vi "Lockin.DAQ.Create Sample Clock.vi"(8 "error in (no error)":errorcluster, 11 "Lockin.DAQ":refnum<class "Instrument.DAQ.lvclass">) -> (0 "error out":errorcluster, 3 "Lockin.DAQ":refnum<class "Instrument.DAQ.lvclass">)   [LabVIEW 2019, in "Instrument.DAQ.lvclass"]
uses:
  Instrument.DAQ.lvclass
  Instrument.DAQ.lvclass/Instrument.DAQ.ctl
  <vilib>/DAQmx/configure/timing.llb/DAQmx Timing (Sample Clock).vi
  <resource>/objmgr/daqmx.rc
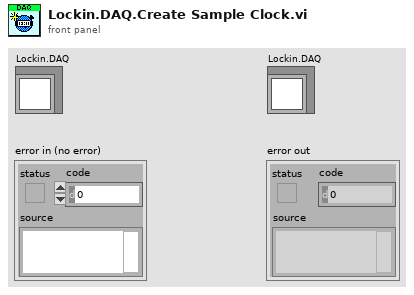
[diagram p1: front panel]
types:
  T1 = typedef "Instrument.DAQ.lvclass/DAQType-enum.ctl" = enum16{"None", "USB 4431", "PXI 446x"}
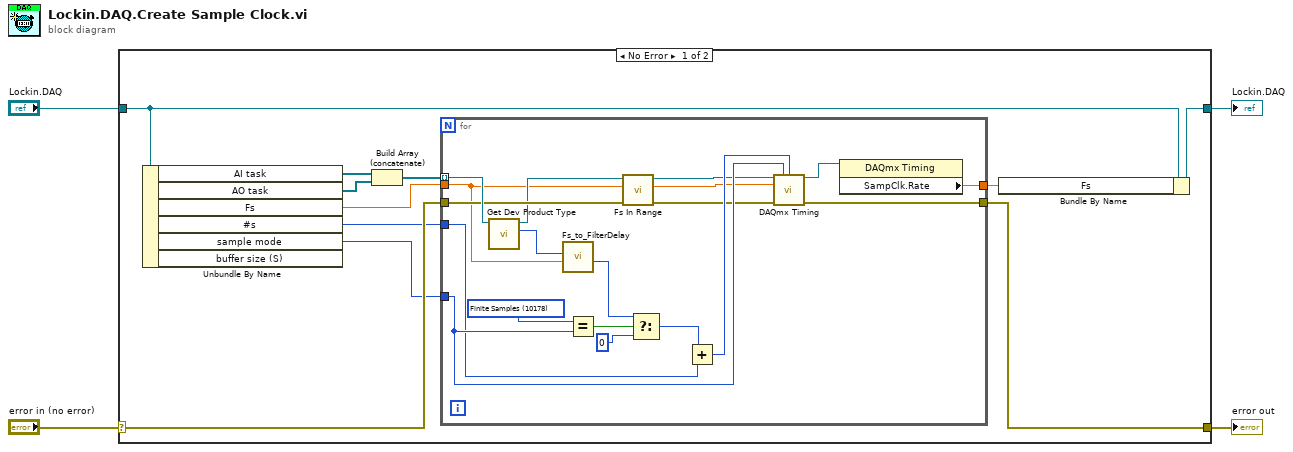
[diagram p0: block diagram]
diagram:
  n1 = case shown="No Error" "error in (no error)" {
    selector: "error in (no error)" -> [w10 w36]
    tunnel: [w11 w36] -> w3
    tunnel: [w6 w35] -> w1
    tunnel: "Lockin.DAQ" -> [w5 w35]
    frame No Error {
      n2 = Unbundle By Name(w5) -> ("AI task"=w15:refnum<k21>[], "AO task"=w14:refnum<k21>[], "Fs"=w12:dbl, "#s"=w9:i32, "sample mode"=w8:i32)  [unwired: 1 out]
      n3 = Build Array (concatenate)(w15, w14) -> (w13:refnum<k21>[])
      n4 = for {
        tunnel: w13 -> [w28] mode=indexing
        tunnel: w12 -> [w23]
        tunnel: w10 -> [w26]
        tunnel: [w34] -> w11
        tunnel: w8 -> [w29]
        tunnel: w9 -> [w17]
        tunnel: [w20] -> w7
        w32 = 10178 items=["Finite Samples"=10178, "Continuous Samples"=10123] ("sample mode 2")
        n5 = call "Get Dev Product Type.vi"("Refnum in"=w28) -> ("DAQ Type"=w27:T1, "Refnum out"=w25:refnum<k21>)  [unwired: 7 in, 2 out]
        n6 = call "Fs_to_FilterDelay.vi"("Fs"=w23, "DAQ Type"=w27) -> ("Total Filter Delay (samples)"=w31:i32)  [unwired: 9 in]
        n7 = Equal?(x=w32, y=w29) -> (x = y?=w33:bool)
        n8 = call "Fs In Range.vi"("error in (no error)"=w26, "Fs"=w23, "Refnum in"=w25) -> ("error out"=w24:errorcluster, "coerced(Fs)"=w21:dbl, "Refnum out"=w19:refnum<k21>)  [unwired: 6 in]
        n9 = Select(t=w31, s=w33, f=0) -> (s? t:f=w16:i32)
        n10 = Add(x=w16, y=w17) -> (x+y=w30:i32)
        n11 = call-poly <vilib>:"DAQmx Timing.vi"("task/channels in"=w19, "sample mode"=w29, "samples per channel"=w30, "rate"=w21, "error in"=w24) -> ("task out"=w22:refnum<k21>, "error out"=w34:errorcluster)  [unwired: 9 in]
        n12 = property class="DAQmx Timing"(reference=w22) -> ("SampClk.Rate"=w20:dbl)  [unwired: 1 in, 2 out]
      }
      n13 = Bundle By Name(cluster=w5, "Fs"=w7) -> (w6:refnum<class "Instrument.DAQ.lvclass">)
    }
    frame Error {
    }
  }
  "error out" <- w3
  "Lockin.DAQ" <- w1
